vi "Transmitter_Example.vi"() -> ()   [LabVIEW 2022 SP3]
uses:
  <instrlib>/niUSRP/niUSRP Write Tx Data (CDB Cluster).vi
panel:
  in  "Alpha":dbl=0.05 min=0.0 max=1.0 step=0.05
  out "Bits length 2":i32
  in  "String 2":string="Hola Mundo! bbbbbbbbbbbbbbbbbbbbbbb\nHola Mundo! bbbbbbbbbbbbbbbbbbbbbbb\nHola Mundo! bbbbbbbbbbbbbbbbbbbbbbb\nHola Mundo! bbbbbbbbbbbbbbbbbbbbbbb"
  in  "Modulation parameter":T1
  out "Bits length":i32
  out "Frame Duration":dbl format="%#_6p"
  out "Waveform Graph":cluster{"t0":dbl, "dt":dbl, "Y":dbl[]}(graph)
  in  "stop":bool
  in  "String":string="Hello World! aaaaaaaaaaaaaaaaaaaaaa\nHello World! aaaaaaaaaaaaaaaaaaaaaa\nHello World! aaaaaaaaaaaaaaaaaaaaaa\nHello World! aaaaaaaaaaaaaaaaaaaaaa"
  out "USRP CoercedParamters":T2={"coerced IQ rate"=100000.0, "coerced carrier frequency"=100000.0, "coerced gain"=0.0} {"coerced gain" format="%#_6f"; "coerced carrier frequency" format="%#_6p"; "coerced IQ rate" format="%#_6p"}
  out "error out":errorcluster
  in  "error in (no error)":errorcluster
  in  "USRP ControledParameters":T3={"active antenna"="TX1", "gain"=0.0, "carrier frequency"=2400000000.0, "IQ rate"=2000000.0} {"IQ rate" format="%#_6p"; "carrier frequency" format="%#_6p"; "gain" format="%#_6f"}
  in  "device names":refnum<k15>="RIO0"
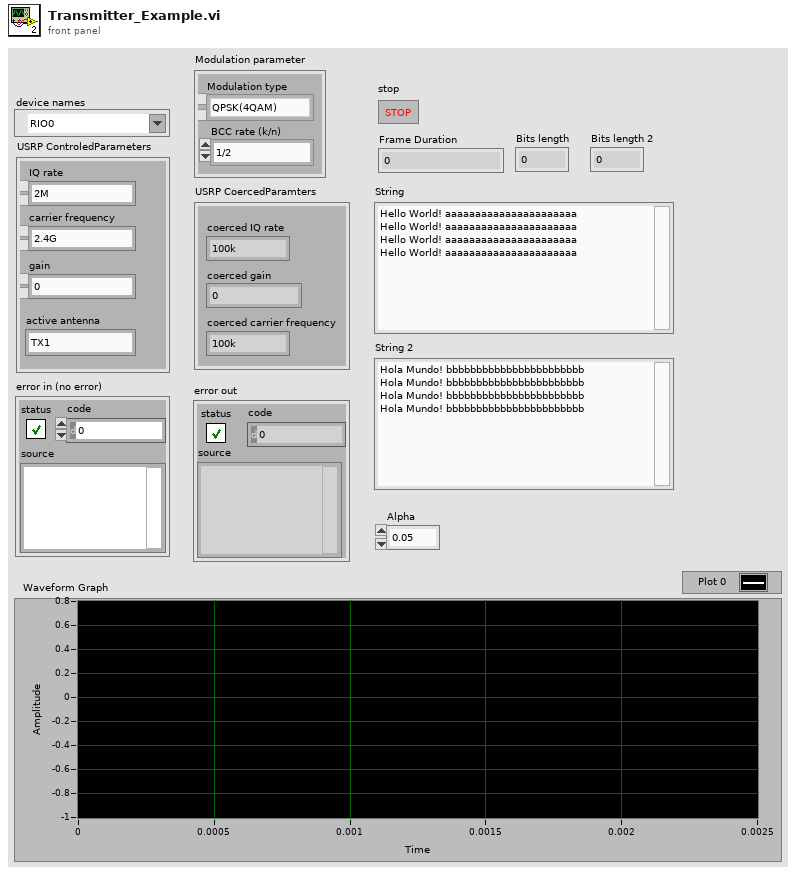
[diagram p1: front panel]
types:
  T1 = cluster{"Modulation type":enum16{"QPSK(4QAM)", "64QAM", "16QAM", "BPSK"}, "BCC rate (k/n)":enum16{"1/2", "2/3", "3/4"}}
  T2 = cluster{"coerced IQ rate":dbl, "coerced carrier frequency":dbl, "coerced gain":dbl}
  T3 = cluster{"active antenna":string, "gain":dbl, "carrier frequency":dbl, "IQ rate":dbl}
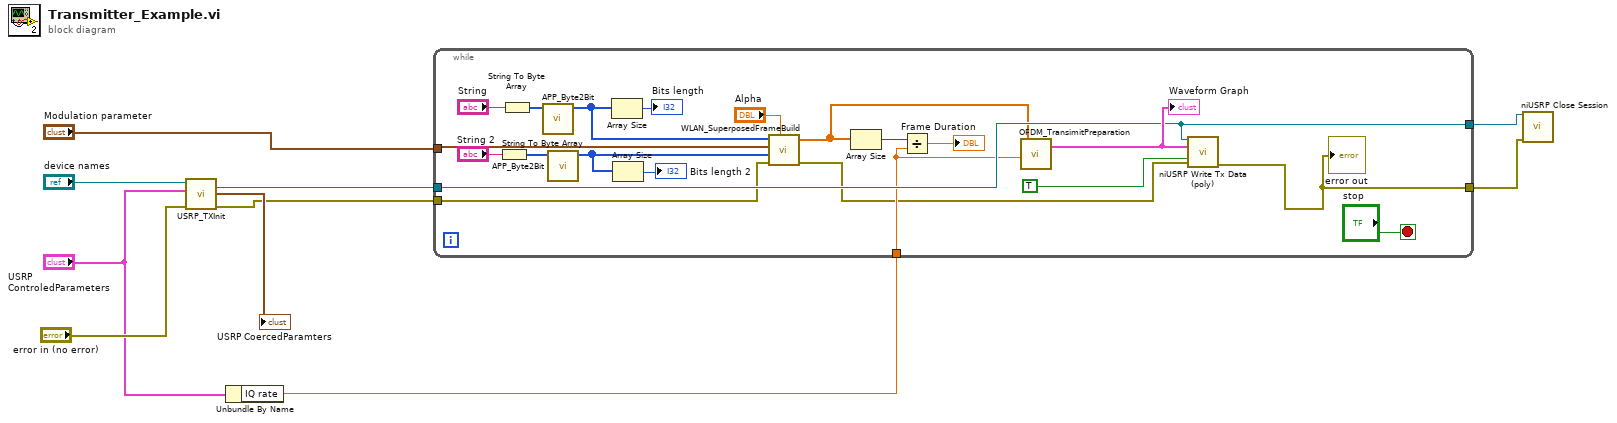
[diagram p0: block diagram]
diagram:
  n1 = call "USRP_TXInit.vi"("device names"="device names", "USRP ControledParameters"="USRP ControledParameters", "error in (no error)"="error in (no error)") -> ("session handle out"=w8:refnum<k15>, "USRP CoercedParamters"=→"USRP CoercedParamters":T2, "error out"=w4:errorcluster)  [unwired: 5 in]
  n2 = Unbundle By Name("USRP ControledParameters") -> ("IQ rate"=w3:dbl)
  n3 = while {
    tunnel: w8 -> [w25]
    tunnel: "Modulation parameter" -> [w16]
    tunnel: w4 -> [w15]
    tunnel: w3 -> [w22]
    tunnel: [w25] -> w2
    tunnel: [w24] -> w1
    stop <- "stop" stop-if-true
    n4 = String To Byte Array(string="String 2") -> (unsigned byte array=w18:u8[])
    n5 = String To Byte Array(string="String") -> (unsigned byte array=w20:u8[])
    n6 = call "APP_Byte2Bit.vi"("input byte stream"=w20) -> ("output bit stream"=w11:i8[])  [unwired: 10 in]
    n7 = call "APP_Byte2Bit.vi"("input byte stream"=w18) -> ("output bit stream"=w17:i8[])  [unwired: 10 in]
    n8 = Array Size(array=w11) -> (size(s)=→"Bits length":i32)
    n9 = Array Size(array=w17) -> (size(s)=→"Bits length 2":i32)
    n10 = call "WLAN_SuperposedFrameBuild.vi"("Alpha"="Alpha", "error in (no error)"=w15, "data in 2"=w17, "Modulation parameter"=w16, "data in"=w11) -> ("error out"=w14:errorcluster, "output array"=w13:cdb[])  [unwired: 5 in]
    n11 = Array Size(array=w13) -> (size(s)=w29:i32)
    n12 = Divide(x=w29, y=w22) -> (x/y=→"Frame Duration":dbl)
    n13 = call "OFDM_TransimitPreparation.vi"("IQ rate"=w22, "array"=w13) -> ("output cluster"=w27:cluster{"t0":dbl, "dt":dbl, "Y":cdb[]})  [unwired: 9 in]
    "Waveform Graph" <- w27
    n14 = call-poly <instrlib>:"niUSRP Write Tx Data (poly).vi"("session handle"=w25, "data"=w27, "end of data?"=TRUE, "error in (no error)"=w14) -> ("error out"=w24:errorcluster)  [unwired: 10 in, 1 out]
    "error out" <- w24
  }
  n15 = call <instrlib>:"niUSRP Close Session.vi"("session handle"=w2, "error in (no error)"=w1) -> ()  [unwired: 13 in, 1 out]
